vi "Pulse_Generator.vi"() -> ()   [LabVIEW 2015]
uses:
  spcm_library/spcm_gui_common.llb/element_device.ctl
  spcm_library/spcm_gui_common.llb/element_pulse_gen_panel.ctl
panel:
  in  "Pulse Gen Panel":T1={"Pulse Gen 0"={"Enable"=TRUE, "Mode"=3, "Len"=100, "High"=50, "Loops"=0, "Delay"=0, "Mux 1"=0, "Mux 2"=1, "Mux1 Invert"=FALSE, "Mux2 Invert"=FALSE, "High Trigger"=FALSE, "Invert Output"=FALSE}, "Pulse Gen 1"={"Enable"=FALSE, "Mode"=3, "Len"=100, "High"=50, "Loops"=0, "Delay"=0, "Mux 1"=0, "Mux 2"=1, "Mux1 Invert"=FALSE, "Mux2 Invert"=FALSE, "High Trigger"=FALSE, "Invert Output"=FALSE}, "Pulse Gen 2"={"Enable"=FALSE, "Mode"=3, "Len"=100, "High"=50, "Loops"=0, "Delay"=0, "Mux 1"=0, "Mux 2"=1, "Mux1 Invert"=FALSE, "Mux2 Invert"=FALSE, "High Trigger"=FALSE, "Invert Output"=FALSE}, "Pulse Gen 3"={"Enable"=FALSE, "Mode"=3, "Len"=100, "High"=50, "Loops"=0, "Delay"=0, "Mux 1"=0, "Mux 2"=1, "Mux1 Invert"=FALSE, "Mux2 Invert"=FALSE, "High Trigger"=FALSE, "Invert Output"=FALSE}} {"Pulse Gen 3"."Mux 2" items=["Unused", "Software", "Card Trigger", "Pulse Gen 0", "Pulse Gen 1", "Pulse Gen 2", "Pulse Gen 3", "XIO 0", "XIO 1", "XIO 2", "XIO 3"]; "Pulse Gen 3"."Mux 1" items=["Unused", "Run", "Arm"]; "Pulse Gen 3"."Mode" items=["Singleshot"=3, "Triggered"=2, "Gated"=1]; "Pulse Gen 2"."Mux 2" items=["Unused", "Software", "Card Trigger", "Pulse Gen 0", "Pulse Gen 1", "Pulse Gen 2", "Pulse Gen 3", "XIO 0", "XIO 1", "XIO 2", "XIO 3"]; "Pulse Gen 2"."Mux 1" items=["Unused", "Run", "Arm"]; "Pulse Gen 2"."Mode" items=["Singleshot"=3, "Triggered"=2, "Gated"=1]; "Pulse Gen 1"."Mux 2" items=["Unused", "Software", "Card Trigger", "Pulse Gen 0", "Pulse Gen 1", "Pulse Gen 2", "Pulse Gen 3", "XIO 0", "XIO 1", "XIO 2", "XIO 3"]; "Pulse Gen 1"."Mux 1" items=["Unused", "Run", "Arm"]; "Pulse Gen 1"."Mode" items=["Singleshot"=3, "Triggered"=2, "Gated"=1]; "Pulse Gen 0"."Mux 2" items=["Unused", "Software", "Card Trigger", "Pulse Gen 0", "Pulse Gen 1", "Pulse Gen 2", "Pulse Gen 3", "XIO 0", "XIO 1", "XIO 2", "XIO 3"]; "Pulse Gen 0"."Mux 1" items=["Unused", "Run", "Arm"]; "Pulse Gen 0"."Mode" items=["Singleshot"=3, "Triggered"=2, "Gated"=1]}
  in  "Start Button":bool
  in  "Quit Button":bool
  in  "Stop Button":bool
  out "Device Infos":T2={"Device Name"="", "Serial Number"=13571.0, "Mem (MB)"=4096.0}
  in  "Device":T3 {"Device" items=["Card", "digitizerNETBOX"]}
  # "Gen3"
  # "Gen2"
  # "Gen1"
  # "Gen0"
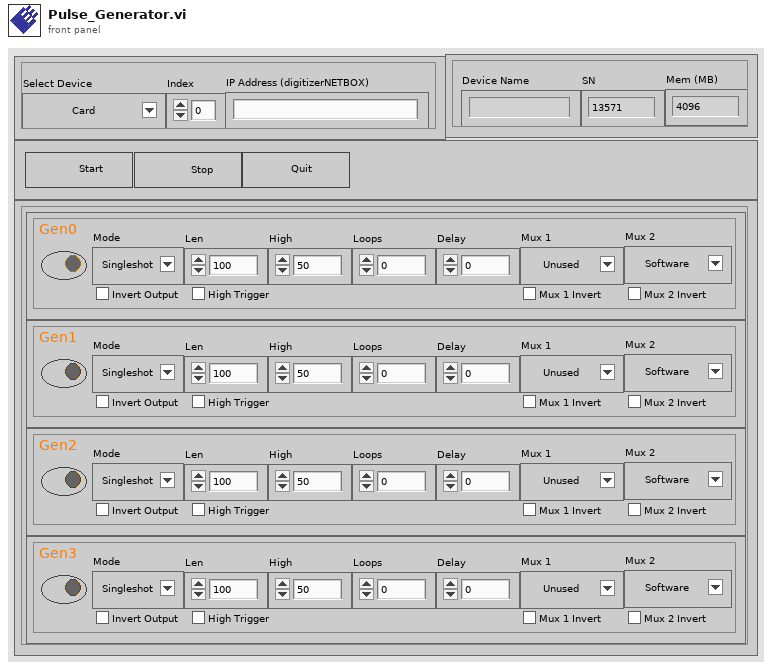
[diagram p1: front panel]
types:
  T1 = typedef "element_pulse_gen_panel.ctl" = cluster{"Pulse Gen 0":cluster{"Enable":bool, "Mode":u16, "Len":i64, "High":i64, "Loops":i64, "Delay":i64, "Mux 1":u16, "Mux 2":u16, "Mux1 Invert":bool, "Mux2 Invert":bool, "High Trigger":bool, "Invert Output":bool}, "Pulse Gen 1":cluster{"Enable":bool, "Mode":u16, "Len":i64, "High":i64, "Loops":i64, "Delay":i64, "Mux 1":u16, "Mux 2":u16, "Mux1 Invert":bool, "Mux2 Invert":bool, "High Trigger":bool, "Invert Output":bool}, "Pulse Gen 2":cluster{"Enable":bool, "Mode":u16, "Len":i64, "High":i64, "Loops":i64, "Delay":i64, "Mux 1":u16, "Mux 2":u16, "Mux1 Invert":bool, "Mux2 Invert":bool, "High Trigger":bool, "Invert Output":bool}, "Pulse Gen 3":cluster{"Enable":bool, "Mode":u16, "Len":i64, "High":i64, "Loops":i64, "Delay":i64, "Mux 1":u16, "Mux 2":u16, "Mux1 Invert":bool, "Mux2 Invert":bool, "High Trigger":bool, "Invert Output":bool}}
  T2 = cluster{"Device Name":string, "Serial Number":dbl, "Mem (MB)":dbl}
  T3 = typedef "element_device.ctl" = cluster{"Index":dbl, "IP Address":string, "Device":u16}
  T4 = enum16{"Idle", "Init", "Write Setup", "Start", "Acquire", "Read Data", "Stop", "Quit"}
  T5 = cluster{"Card Type":i32, "Inst Mem (high part)":i32, "Inst Mem (low part)":i32, "Serial Number":i32, "Function Type":i32, "Installed Features":i32, "Base Card Version":i32, "Module Version":i32, "Extension Version":i32, "Production Date":i32, "Max Sampling Rate":i32, "Max Channels":i32, "Demo Card":i32}
  T6 = cluster{"Card Name":string, "SN":i32, "Mem (MB)":i32}
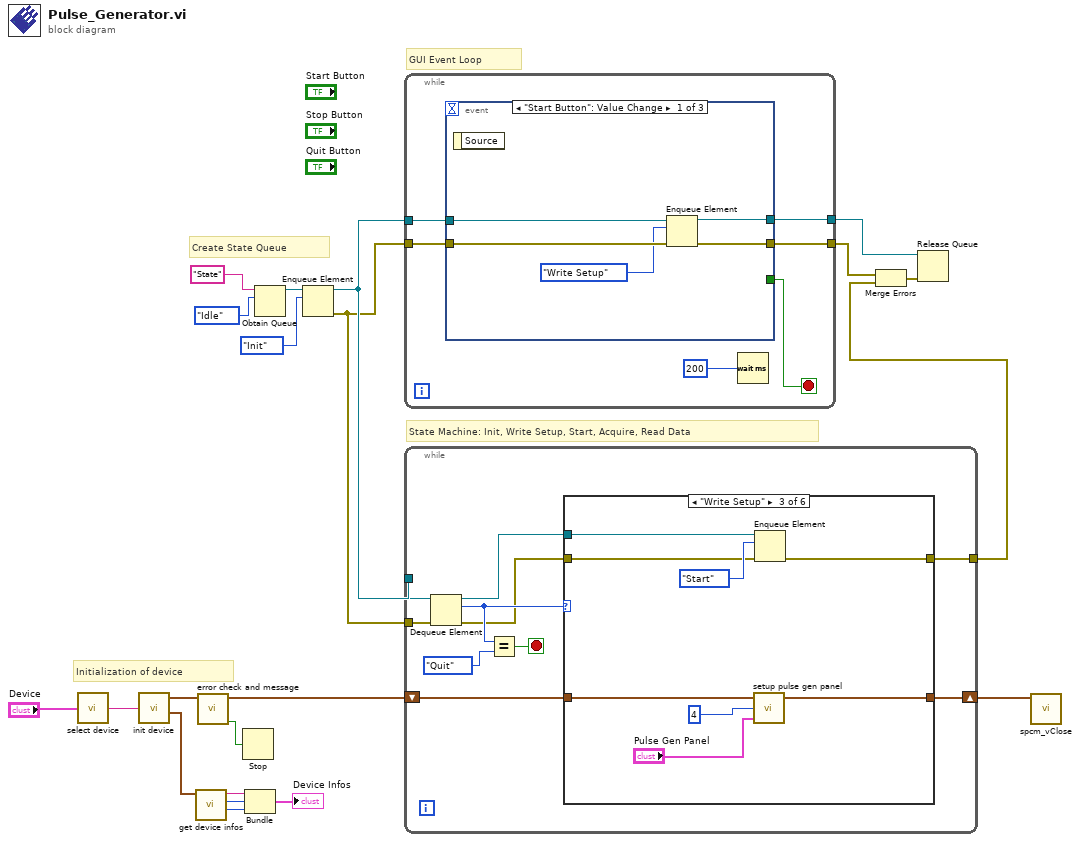
[diagram p0: block diagram]
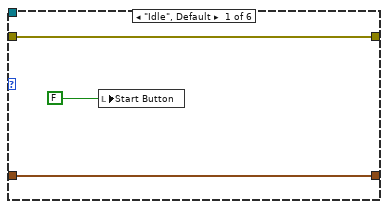
[diagram p2: hidden frame]
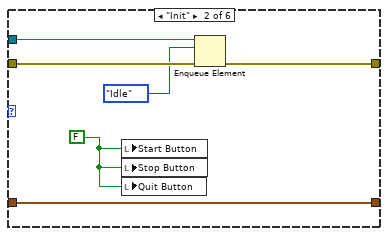
[diagram p3: hidden frame]
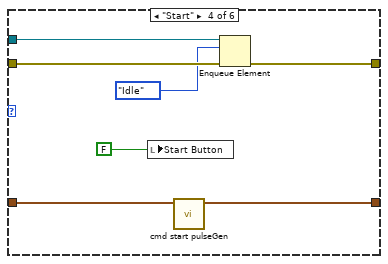
[diagram p4: hidden frame]
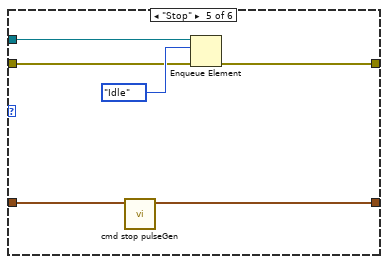
[diagram p5: hidden frame]
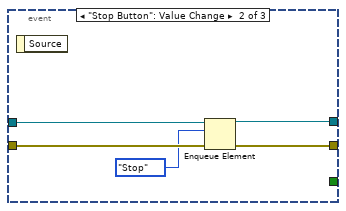
[diagram p7: hidden frame]
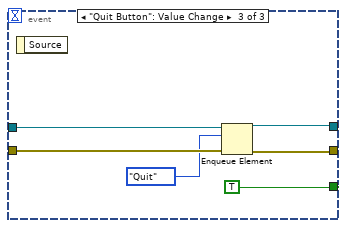
[diagram p8: hidden frame]
diagram:
  # "Initialization of device"
  # "Create State Queue"
  # "State Machine: Init, Write Setup, Start, Acquire, Read Data"
  # "GUI Event Loop"
  n1 = call "select device.vi"("Device"="Device") -> ("device string"=w21:string)  [unwired: 4 in]
  n2 = call "init device.vi"("Device String"=w21) -> ("Card Info Out"=w20:cluster{"Card Handle":u64, "Error Code":u32}, "Card Information"=w9:T5)  [unwired: 4 in]
  n3 = call "get device infos.vi"("Card Information"=w9) -> ("Mem (MB)"=w13:i32, "SN"=w12:i32, "Card Name"=w11:string)  [unwired: 8 in]
  n4 = call "error check and message.vi"("Card Info In"=w20) -> ("Error occurred"=w19:bool, "Card Info Out"=w1:cluster{"Card Handle":u64, "Error Code":u32})  [unwired: 4 in, 1 out]
  n5 = Stop(stop? (T)=w19) -> ()
  n6 = Bundle("Card Name"=w11, "SN"=w12, "Mem (MB)"=w13) -> (→"Device Infos":T6)  [unwired: 1 in]
  n7 = Obtain Queue(name (unnamed)="State", element data type=T4."Idle") -> (queue out=w16:refnum<queue>)  [unwired: 3 in, 2 out]
  n8 = Enqueue Element(queue=w16, element=T4."Init") -> (queue out=w17:refnum<queue>, error out=w4:errorcluster)  [unwired: 2 in, 1 out]
  n9 = while {
    tunnel: w17 -> [w25]
    tunnel: [w26] -> w5
    tunnel: [w22] -> w8
    tunnel: w4 -> [w23]
    stop <- w24 stop-if-true
    n10 = event shown="[0] \"Start Button\": Value Change" {
      selector: _ -> [_ _ _]
      dyn-events: _ -> [_ _ _]
      timeout: _ -> [_ _ _]
      tunnel: [_ _ TRUE] -> w24
      tunnel: [w32 w37 w42] -> w26
      tunnel: w25 -> [w31 w36 w43]
      tunnel: [w29 w34 w40] -> w22
      tunnel: w23 -> [w30 w35 w39]
      event "Start Button": Value Change {
        n11 = event-data() -> ()  [unwired: 1 in, 1 out]
        n12 = Enqueue Element(queue=w31, element=T4."Write Setup", error in (no error)=w30) -> (queue out=w32:refnum<queue>, error out=w29:errorcluster)  [unwired: 1 in, 1 out]
      }
      event "Stop Button": Value Change {
        n13 = event-data() -> ()  [unwired: 1 in, 1 out]
        n14 = Enqueue Element(queue=w36, element=T4."Stop", error in (no error)=w35) -> (queue out=w37:refnum<queue>, error out=w34:errorcluster)  [unwired: 1 in, 1 out]
      }
      event "Quit Button": Value Change {
        n15 = event-data() -> ()  [unwired: 1 in, 1 out]
        n16 = Enqueue Element(queue=w43, element=T4."Quit", error in (no error)=w39) -> (queue out=w42:refnum<queue>, error out=w40:errorcluster)  [unwired: 1 in, 1 out]
      }
    }
    n17 = Wait (ms)(milliseconds to wait=200) -> ()  [unwired: 1 out]
  }
  n18 = while {
    tunnel: w17 -> [w53]
    shift-right: [w51] -> w15
    shift-left: w1 -> [w52]
    tunnel: [w47] -> w7
    tunnel: w4 -> [w46]
    stop <- w49 stop-if-true
    n19 = Dequeue Element(queue=w53, error in (no error)=w46) -> (queue out=w48:refnum<queue>, element=w50:T4, error out=w45:errorcluster)  [unwired: 1 in, 1 out]
    n20 = Equal?(x=w50, y=T4."Quit") -> (x = y?=w49:bool)
    n21 = case shown="\"Write Setup\"" w50 {
      tunnel: w52 -> [w56 w58 w66 w72 w79 w84]
      tunnel: [w56 w58 w65 w71 w78 w84] -> w51
      tunnel: w48 -> [_ w62 w68 w76 w81 _]
      tunnel: [w55 w61 w70 w75 w83 w85] -> w47
      tunnel: w45 -> [w55 w60 w67 w77 w80 w85]
      frame "Idle", Default {
        n22 = local write "Start Button"(FALSE) -> ()
      }
      frame "Init" {
        w57 = FALSE
        n23 = local write "Start Button"(w57) -> ()
        n24 = local write "Stop Button"(w57) -> ()
        n25 = local write "Quit Button"(w57) -> ()
        n26 = Enqueue Element(queue=w62, element=T4."Idle", error in (no error)=w60) -> (error out=w61:errorcluster)  [unwired: 1 in, 2 out]
      }
      frame "Write Setup" {
        n27 = call "setup pulse gen panel.vi"("Pulse Gen Panel"="Pulse Gen Panel", "Num Pulse Gen"=4, "Card Info In"=w66) -> ("Card Info Out"=w65:cluster{"Card Handle":u64, "Error Code":u32})  [unwired: 2 in]
        n28 = Enqueue Element(queue=w68, element=T4."Start", error in (no error)=w67) -> (error out=w70:errorcluster)  [unwired: 1 in, 2 out]
      }
      frame "Start" {
        n29 = local write "Start Button"(FALSE) -> ()
        n30 = call "cmd start pulseGen.vi"("Card Info In"=w72) -> ("Card Info Out"=w71:cluster{"Card Handle":u64, "Error Code":u32})  [unwired: 6 in]
        n31 = Enqueue Element(queue=w76, element=T4."Idle", error in (no error)=w77) -> (error out=w75:errorcluster)  [unwired: 1 in, 2 out]
      }
      frame "Stop" {
        n32 = call "cmd stop pulseGen.vi"("Card Info In"=w79) -> ("Card Info Out"=w78:cluster{"Card Handle":u64, "Error Code":u32})  [unwired: 6 in]
        n33 = Enqueue Element(queue=w81, element=T4."Idle", error in (no error)=w80) -> (error out=w83:errorcluster)  [unwired: 1 in, 2 out]
      }
      frame "Quit" {
      }
    }
  }
  n34 = Merge Errors(w8, w7) -> (w6:errorcluster)
  n35 = Release Queue(queue=w5, error in (no error)=w6) -> ()  [unwired: 1 in, 3 out]
  n36 = call "spcm_vClose.vi"("Card Info In"=w15) -> ()  [unwired: 7 in]
